vi "HumanFancyDrive.vi"(10 "X Axis":dbl, 11 "Y Axis":dbl) -> (2 "Right Motor Value":dbl, 3 "Left Motor Value":dbl)   [LabVIEW 2020]
doc: "A modified arcade drive that makes the robot drive good."
uses:
  <vilib>/Rock Robotics/WPI/ThirdParty/JAS_Junk/TrajLib/Trajectory_Library.lvlib
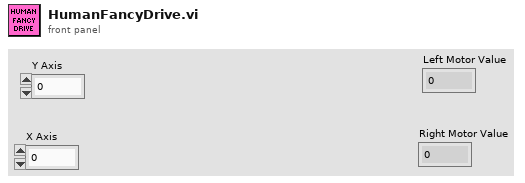
[diagram p1: front panel]
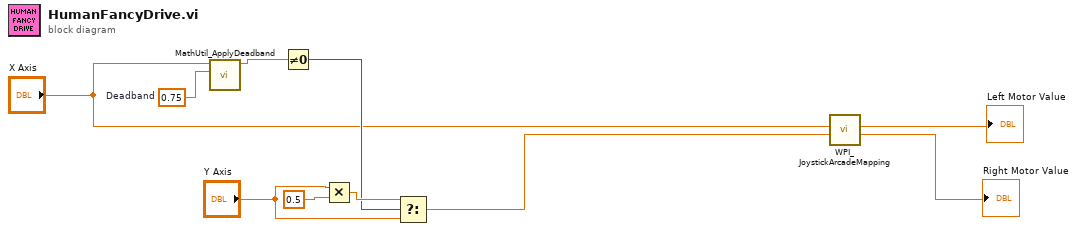
[diagram p0: block diagram]
diagram:
  w8 = 0.75  # Deadband
  n1 = call <vilib>:"MathUtil_ApplyDeadband.vi"("Deadband"=w8, "Value"="X Axis") -> ("Result"=w6:dbl)  [unwired: 9 in]
  n2 = Not Equal To 0?(x=w6) -> (x != 0?=w5:bool)
  n3 = Multiply(x="Y Axis", y=0.5) -> (x*y=w10:dbl)
  n4 = Select(t=w10, s=w5, f="Y Axis") -> (s? t:f=w3:dbl)
  n5 = call <vilib>:"WPI_JoystickArcadeMapping.vi"("Y axis value"=w3, "X axis value"="X Axis") -> ("Right Motor Value"=→"Right Motor Value":dbl, "Left Motor Value"=→"Left Motor Value":dbl)  [unwired: 8 in]
